vi "OCR_MakeTrainedData.vi"(8 "error in (no error)":errorcluster, 10 "exp#":string, 11 "lang.font.exp":string) -> (0 "error out":errorcluster, 2 "standard error":string[](array[string]), 3 "standard output":string[](array[string]))   [LabVIEW 2019]
uses:
  Controls/cmd.ctl
panel:
  out "error":bool
  # "eng1.segoe.exp1.tr"
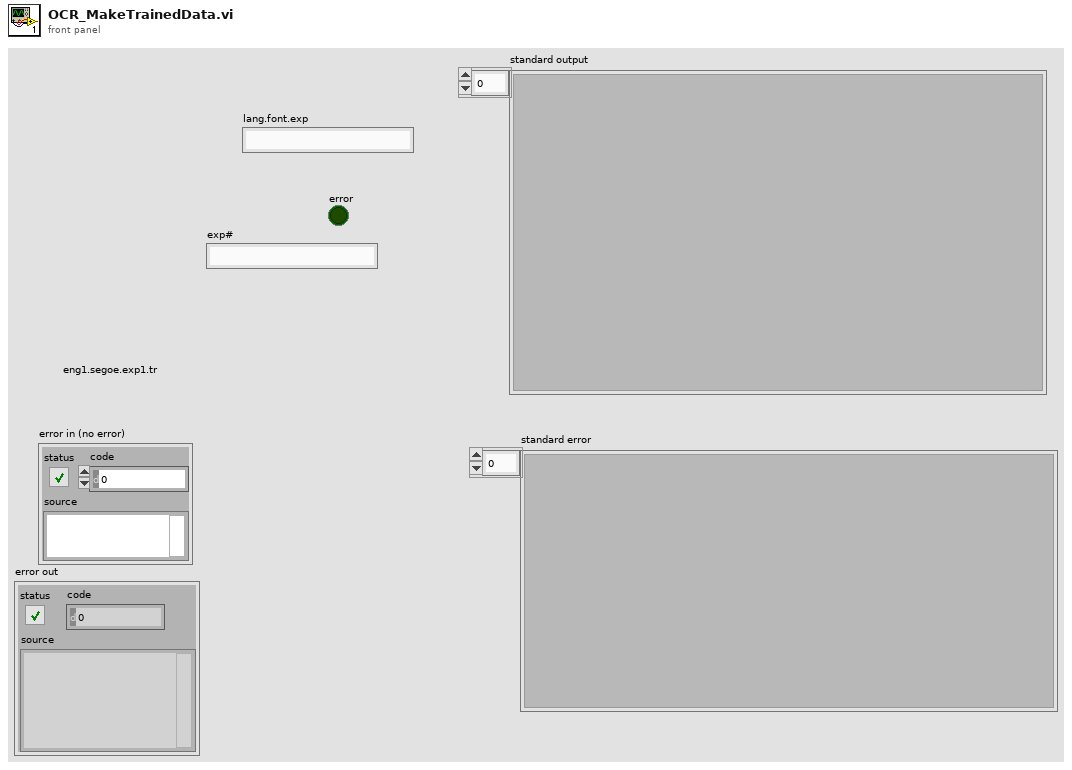
[diagram p1: front panel]
types:
  T1 = typedef "cmd.ctl" = enum16{"Box Train", "unicharset", "ShapeTable", "mftraining1", "mftraining2", "cntraining", "rename", "move files", "combine"}
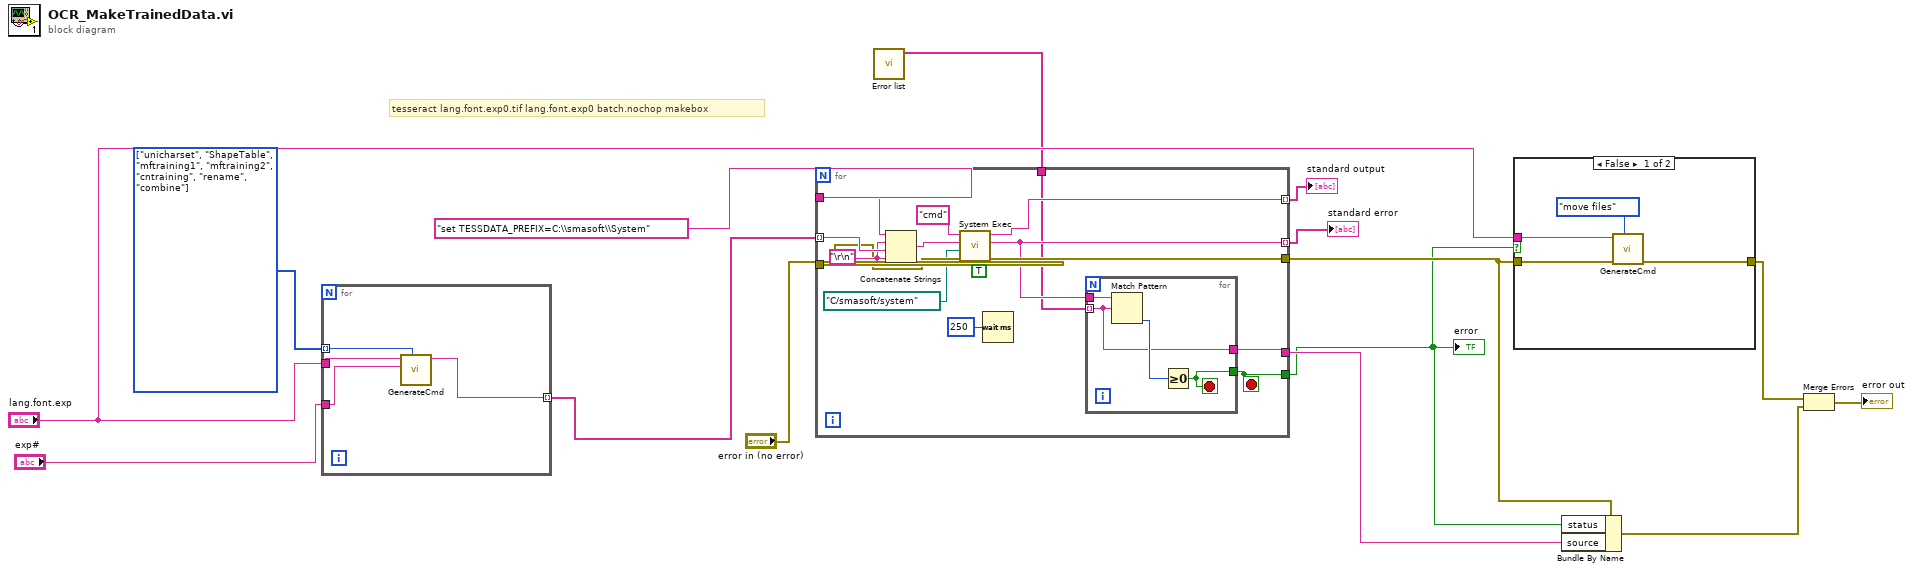
[diagram p0: block diagram]
diagram:
  w15 = T1[] [enum."unicharset", enum."ShapeTable", enum."mftraining1", enum."mftraining2", enum."cntraining", enum."rename", enum."combine"] items=["Box Train", "unicharset", "ShapeTable", "mftraining1", "mftraining2", "cntraining", "rename", "move files", "combine"] ("Array")
  # "tesseract lang.font.exp0.tif lang.font.exp0 batch.nochop makebox"
  n1 = for {
    tunnel: w15 -> [w19] mode=indexing
    tunnel: "lang.font.exp" -> [w18]
    tunnel: "exp#" -> [w17]
    tunnel: [w16] -> w9 mode=indexing
    n2 = call "GenerateCmd.vi"("Cmd"=w19, "exp#"=w17, "lang.font.exp"=w18) -> ("CMD"=w16:string)  [unwired: 7 in, 1 out]
  }
  n3 = call "Error list.vi"() -> ("regular expression"=w3:string[])  [unwired: 11 in]
  n4 = for {
    tunnel: w9 -> [w34] mode=indexing
    tunnel: "set TESSDATA_PREFIX=C:\\smasoft\\System" ("standard input") -> [w32]
    tunnel: "error in (no error)" -> [w27]
    tunnel: [w26] -> w7
    tunnel: [w23] -> w4 mode=indexing
    tunnel: [w24] -> w5 mode=indexing
    tunnel: w3 -> [w22]
    tunnel: [w21] -> w2
    tunnel: [w20] -> w1
    stop <- w20 stop-if-true
    w33 = "\r\n"
    n5 = Concatenate Strings(w32, w33, w34, w33) -> (w31:string)
    n6 = call <vilib>:"System Exec.vi"("run minimized? (F)"=TRUE, "error in (no error)"=w27, "working directory"=path "C:/smasoft/system", "standard input"=w31, "command line"="cmd") -> ("error out"=w26:errorcluster, "standard error"=w23:string, "standard output"=w24:string)  [unwired: 3 in, 1 out]
    n7 = Wait (ms)(milliseconds to wait=u32 250) -> ()  [unwired: 1 out]
    n8 = for {
      tunnel: w23 -> [w37]
      tunnel: w22 -> [w36] mode=indexing
      tunnel: [w36] -> w21
      tunnel: [w35] -> w20
      stop <- w35 stop-if-true
      n9 = Match Pattern(string=w37, regular expression=w36) -> (offset past match=w38:i32)  [unwired: 1 in, 3 out]
      n10 = Greater Or Equal To 0?(x=w38) -> (x >= 0?=w35:bool)
    }
  }
  "error" <- w1
  "standard output" <- w5
  "standard error" <- w4
  n11 = case shown="False" w1 {
    tunnel: w7 -> [w42 _]
    tunnel: "lang.font.exp" -> [w41 _]
    tunnel: [w40 _] -> w12
    frame False {
      n12 = call "GenerateCmd.vi"("Cmd"=cmd."move files", "error in"=w42, "lang.font.exp"=w41) -> ("error Out"=w40:errorcluster)  [unwired: 7 in, 1 out]
    }
    frame True {
    }
  }
  n13 = Bundle By Name(cluster=w7, "status"=w1, "source"=w2) -> (w11:errorcluster)
  n14 = Merge Errors(w12, w11) -> (→"error out":errorcluster)
